vi "RELAYS Read the Baudrate.vi"(8 "error in (no error)":errorcluster, 10 "Dev addr":u8=1 format="%x", 11 "VISA resource name":refnum<visa-resource-name>) -> (0 "error out":errorcluster, 1 "baudrate":T1=3 items=["4800"=2, "9600"=3, "19200"=4], 2 "ack":string, 3 "VISA resource name out":refnum<visa-resource-name>)   [LabVIEW 2016, in "MB _relays.lvlib"]
uses:
  MB _relays.lvlib
  type defs/baudrate.ctl
  private/gen MB frame -Get the Baudrate.vi
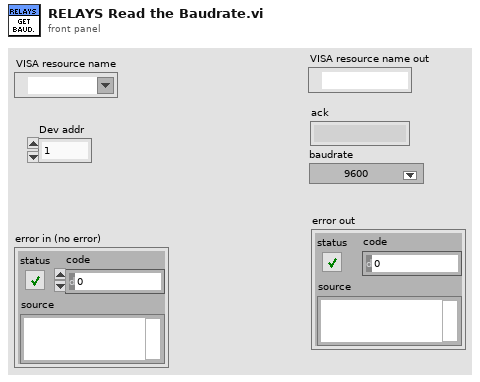
[diagram p1: front panel]
types:
  T1 = typedef "MB _relays.lvlib/baudrate.ctl" = u8
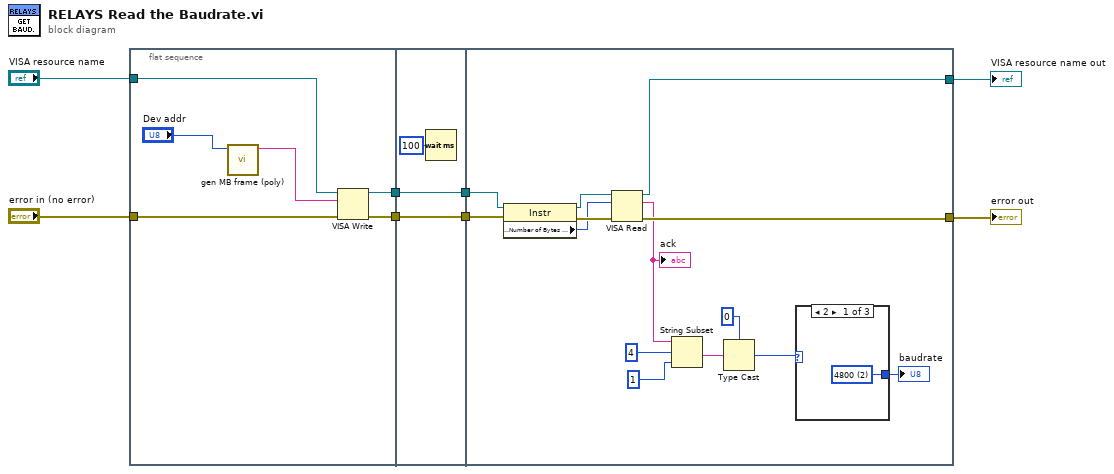
[diagram p0: block diagram]
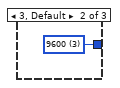
[diagram p2: hidden frame]
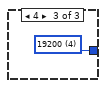
[diagram p3: hidden frame]
diagram:
  n1 = flat-sequence {
    tunnel: "error in (no error)" -> [w11]
    tunnel: "VISA resource name" -> [w10]
    tunnel: [w14] -> w4
    tunnel: [w13] -> w3
    tunnel: w4 -> [w17]
    tunnel: w3 -> [w16]
    tunnel: [w17] -> w2
    tunnel: [w16] -> w1
    tunnel: [w25] -> w7
    tunnel: [w26] -> w8
    tunnel: w2 -> [w30]
    tunnel: w1 -> [w31]
    frame #0 {
      n2 = call-poly "gen MB frame (poly).vi"("Dev Addr"="Dev addr") -> ("MB frame"=w12:string)  [unwired: 10 in]
      n3 = VISA Write(VISA resource name=w10, write buffer=w12, error in (no error)=w11) -> (VISA resource name out=w14:refnum<visa-resource-name>, error out=w13:errorcluster)  [unwired: 1 out]
    }
    frame #1 {
      n4 = Wait (ms)(milliseconds to wait=u32 100) -> ()  [unwired: 1 out]
    }
    frame #2 {
      n5 = property class="Instr"(reference=w30, error in=w31) -> (reference out=w28:refnum<visa-resource-name>, error out=w29:errorcluster, "Serial Settings:Number of Bytes at Serial Port"=w27:u32)
      n6 = VISA Read(VISA resource name=w28, byte count=w27, error in (no error)=w29) -> (VISA resource name out=w26:refnum<visa-resource-name>, read buffer=w24:string, error out=w25:errorcluster)  [unwired: 1 out]
      "ack" <- w24
      n7 = String Subset(string=w24, offset (0)=4, length (rest)=1 ("length (rest)")) -> (substring=w21:string)
      n8 = Type Cast(type=u8 0, x=w21) -> (*(type *) &x=w19:u8)
      n9 = case shown="2" w19 {
        tunnel: [w32 w33 w34] -> w18
        frame 2 {
          w32 = T1 2 items=["4800"=2, "9600"=3, "19200"=4] ("baudrate")
        }
        frame 3, Default {
          w33 = T1 3 items=["4800"=2, "9600"=3, "19200"=4] ("baudrate")
        }
        frame 4 {
          w34 = T1 4 items=["4800"=2, "9600"=3, "19200"=4] ("baudrate")
        }
      }
      "baudrate" <- w18
    }
  }
  "VISA resource name out" <- w8
  "error out" <- w7
